vi "convertToKeyValuePair_string.vi"(8 "error in (no error)":errorcluster, 9 "double quotes (T)":bool=TRUE, 10 "value":string, 11 "name":string) -> (0 "error out":errorcluster, 3 "string converted":string)   [LabVIEW 2018]
doc: "Convert a string into a key value pair as string."
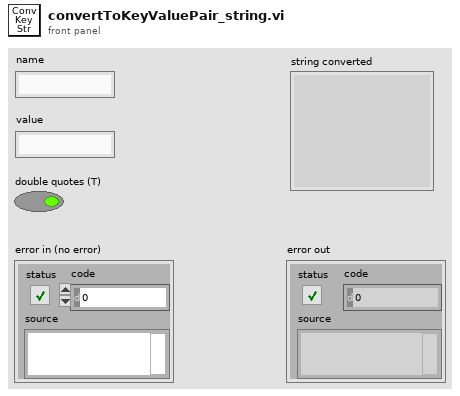
[diagram p1: front panel]
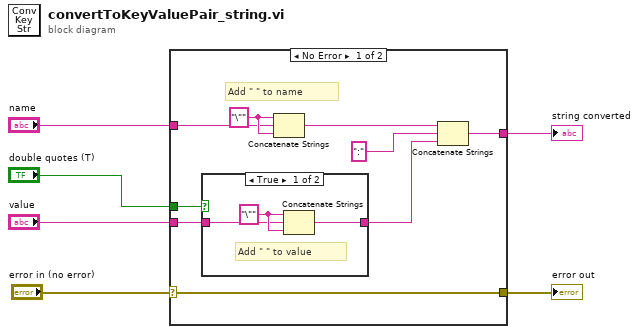
[diagram p0: block diagram]
diagram:
  n1 = case shown="No Error" "error in (no error)" {
    selector: "error in (no error)" -> [w10 w20]
    tunnel: [w15 _] -> w6
    tunnel: "name" -> [w13 _]
    tunnel: [w10 w20] -> w3
    tunnel: "value" -> [w9 _]
    tunnel: "double quotes (T)" -> [w7 _]
    frame No Error {
      w14 = "\"" ("string")
      # "Add \" \" to name"
      n2 = case shown="True" w7 {
        tunnel: w9 -> [w17 w19]
        tunnel: [w16 w19] -> w8
        frame True {
          w18 = "\"" ("string")
          # "Add \" \" to value"
          n3 = Concatenate Strings(w18, w17, w18) -> (w16:string)
        }
        frame False {
        }
      }
      n4 = Concatenate Strings(w14, w13, w14) -> (w12:string)
      n5 = Concatenate Strings(w12, ":" ("string"), w8) -> (w15:string)
    }
    frame Error {
    }
  }
  "error out" <- w3
  "string converted" <- w6
